vi "A33ConfigureFM_py.vi"(8 "error in (no error)":errorcluster, 10 "Instrument":string, 11 "socket in":refnum<class "zmq_socket.lvclass">) -> (0 "error out":errorcluster, 1 "Standalone":bool, 2 "resulting string":string, 3 "socket out":refnum<class "zmq_socket.lvclass">)   [LabVIEW 2022 SP3]
doc: "Selects the waveform shape, frequency, amplitude, offset, and phase for a standard waveform."
uses:
  <vilib>/addons/zeromq/zmq_socket.lvclass
panel:
  in  "FM Source (0: Internal)":i32(ring) items=["Internal", "External", "Channel 1", "Channel 2"]
  in  "Modulation Waveform (0: Sine)":i32(ring) items=["Sine", "Square", "Triangle", "Ramp", "Negative Ramp", "Noise", "PRBS", "ARB"]
  in  "Channel (1: Channel1)":i32(ring)=1 items=["Channel1"=1, "Channel2"=2]
  in  "Enable Frequency Modulation (T:Enable)":bool=TRUE
  in  "Modulation Deviation (100.0 Hz)":dbl=100.0 format="%#_12g"
  in  "Modulation Frequency (1000.0 Hz)":dbl=1000.0 format="%#_12g"
  # "Min 1uHz, Max 60 MHz"
  # "Min 1uHz to max for this WFM\nMax for TRIAG - 800 kHz"
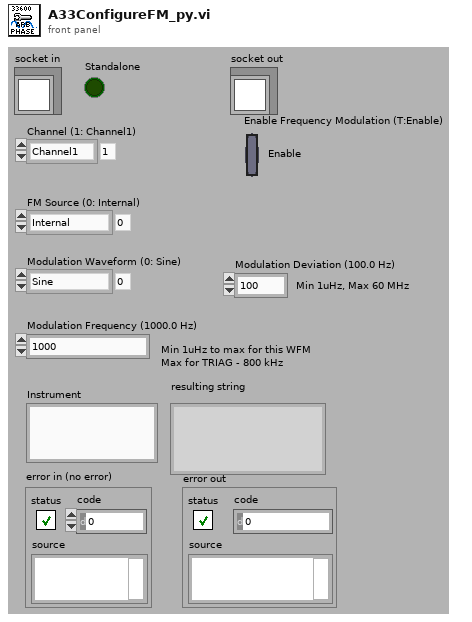
[diagram p1: front panel]
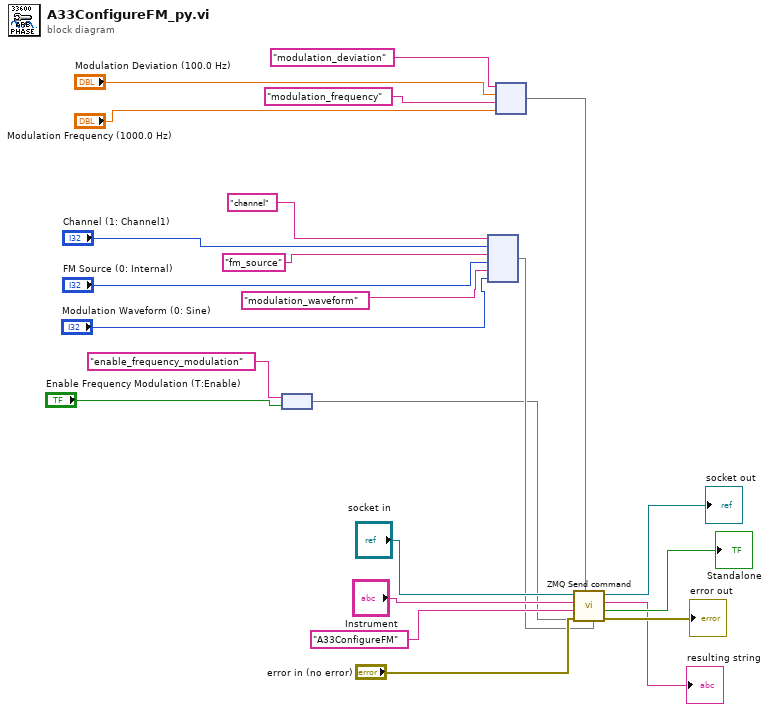
[diagram p0: block diagram]
diagram:
  n1 = node("enable_frequency_modulation" ("key"), "Enable Frequency Modulation (T:Enable)") -> (w6:map{string, bool})
  n2 = node("channel" ("key"), "Channel (1: Channel1)", "fm_source" ("key"), "FM Source (0: Internal)", "modulation_waveform" ("key"), "Modulation Waveform (0: Sine)") -> (w14:map{string, i32})
  n3 = node("modulation_deviation" ("key"), "Modulation Deviation (100.0 Hz)", "modulation_frequency" ("key"), "Modulation Frequency (1000.0 Hz)") -> (w1:map{string, dbl})
  n4 = call "ZMQ Send command.vi"("Int args"=w14, "Bool args"=w6, "DBL args"=w1, "error in"="error in (no error)", "Command"="A33ConfigureFM", "Instrument"="Instrument", "socket in"="socket in") -> ("error out"=→"error out":errorcluster, "Standalone"=→"Standalone":bool, "Recieved message"=→"resulting string":string, "socket out"=→"socket out":refnum<class "zmq_socket.lvclass">)  [unwired: 1 in]
